vi "Aircraft Offline.vi"(8 "Error In":errorcluster, 11 "Aircraft ID":u8) -> (0 "Error Out":errorcluster)   [LabVIEW 2014]
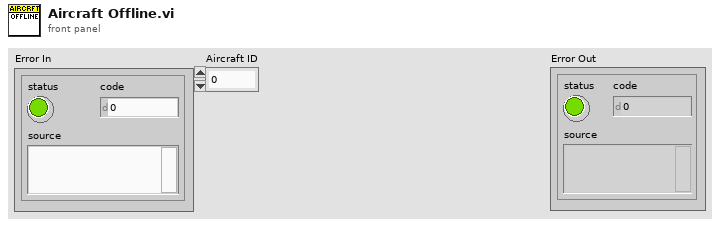
[diagram p1: front panel]
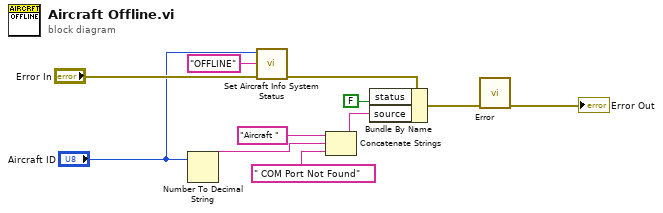
[diagram p0: block diagram]
diagram:
  n1 = Number To Decimal String(number="Aircraft ID") -> (decimal integer string=w9:string)  [unwired: 1 in]
  n2 = call "Set Aircraft Info System Status.vi"("Error In"="Error In", "System Status"="OFFLINE", "Aircraft ID"="Aircraft ID") -> ("Error Out"=w6:errorcluster)  [unwired: 8 in]
  n3 = Concatenate Strings("Aircraft " ("string"), w9, " COM Port Not Found" ("string")) -> (w7:string)
  n4 = Bundle By Name(cluster=w6, "status"=FALSE, "source"=w7) -> (w4:errorcluster)
  n5 = call "Error.vi"("Error In"=w4) -> ("Error Out"=→"Error Out":errorcluster)  [unwired: 10 in]
